vi "WPI_CameraSet White Balance.vi"(8 "error in (no error)":errorcluster, 9 "Color Temp (K)":dbl, 10 "White Balance":T2, 11 "CameraDevRef":T1={"Camera Address"="192.168.0.90", "CameraStatus"={"status"=FALSE, "code"=0, "source"=""}}) -> (0 "error out":errorcluster, 3 "CameraDevRef Out":T1)   [LabVIEW 2017]
doc: "Specifies the white balance setting of the camera you specify.\n\nThis software is licensed. Open the labview\\readme\\WPI Robotics Library Open Source License.txt file for more information."
uses:
  <vilib>/Rock Robotics/WPI/Camera/WPI_CameraWhite Balance Values.ctl
  <vilib>/Rock Robotics/WPI/Camera/WPI_CameraDevRef.ctl
  <vilib>/Rock Robotics/WPI/Camera/WPI_CameraSettings Operations.ctl
  <vilib>/userdefined/High Color/IMAQdx.ctl
  <resource>/objmgr/imaqdx.rc
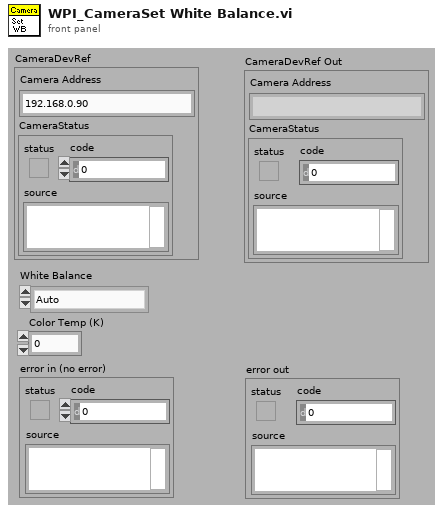
[diagram p1: front panel]
types:
  T1 = typedef "WPI_CameraDevRef.ctl" = cluster{"Camera Address":string, "CameraStatus":errorcluster}
  T2 = typedef "WPI_CameraWhite Balance Values.ctl" = enum16{"Auto", "Fixed indoor", "Fixed outdoor 1", "Fixed outdoor 2", "Fixed fluorescent 1", "Fixed fluorescent 2", "Hold current", "Custom"}
  T3 = typedef "WPI_CameraSettings Operations.ctl" = enum16{"Udate FPS", "Update Compression", "Update Size", "Update White Balance", "Update Brightness", "Update Sharpness", "Update Exposure", "Update Exposure Value", "Update Color Level", "Update Exp Priority", "Update Color Enable", "Update JPG", "Update MJPG", "Read and Clear", "Read", "Init"}
  T4 = typedef "IMAQdx.ctl" = refnum<k21>
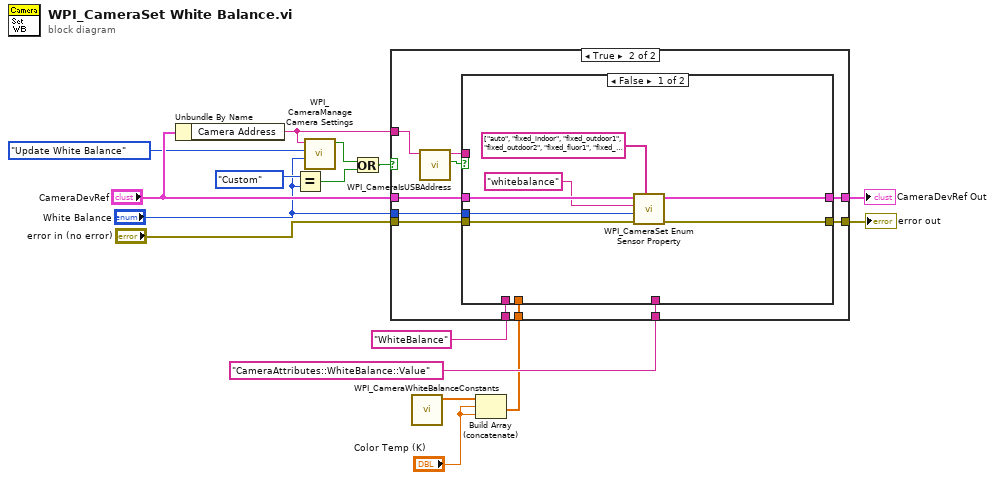
[diagram p0: block diagram]
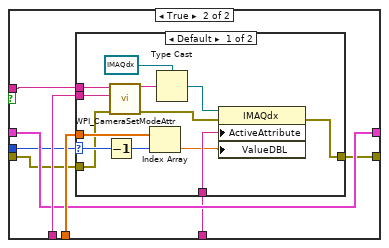
[diagram p3: hidden frame]
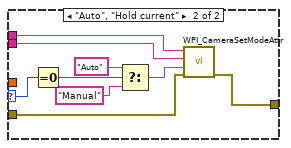
[diagram p4: hidden frame]
diagram:
  n1 = Unbundle By Name("CameraDevRef") -> ("Camera Address"=w11:string)
  n2 = Equal?(x=WPI_CameraWhite_Balance_Values."Custom" ("White Balance"), y="White Balance") -> (x = y?=w3:bool)
  n3 = call <vilib>:"WPI_CameraManage Camera Settings.vi"("Value"="White Balance", "Operation"=WPI_CameraSettings_Operations."Update White Balance", "Camera IP"=w11) -> ("Changed"=w2:bool)  [unwired: 7 in, 1 out]
  n4 = Or(x=w2, y=w3) -> (x .or. y?=w1:bool)
  n5 = call <vilib>:"WPI_CameraWhiteBalanceConstants.vi"() -> ("Color Temps (K)"=w8:dbl[])  [unwired: 11 in]
  n6 = Build Array (concatenate)(w8, "Color Temp (K)", "Color Temp (K)") -> (w7:dbl[])
  n7 = case shown="True" w1 {
    tunnel: [w18 w29] -> w16
    tunnel: [w17 w28] -> w15
    tunnel: "error in (no error)" -> [w17 w27]
    tunnel: "CameraDevRef" -> [w18 w25]
    tunnel: "White Balance" -> [_ w26]
    tunnel: w11 -> [_ w22]
    tunnel: "WhiteBalance" -> [_ w21]
    tunnel: w7 -> [_ w20]
    tunnel: "CameraAttributes::WhiteBalance::Value" -> [_ w19]
    frame False {
    }
    frame True {
      n8 = call <vilib>:"WPI_CameraIsUSBAddress.vi"("Camera Address In"=w22) -> ("USB?"=w24:bool, "Camera Address Out"=w23:string)  [unwired: 8 in, 1 out]
      n9 = case shown="False" w24 {
        tunnel: [w36 w42] -> w29
        tunnel: [w35 w37] -> w28
        tunnel: w27 -> [w34 w38]
        tunnel: w26 -> [w33 w41]
        tunnel: w25 -> [w32 w42]
        tunnel: w23 -> [_ w39]
        tunnel: w21 -> [_ w44]
        tunnel: w20 -> [_ w43]
        tunnel: w19 -> [_ w40]
        frame False {
          n10 = call <vilib>:"WPI_CameraSet Enum Sensor Property.vi"("Strings"=string[] ["auto", "fixed_indoor", "fixed_outdoor1", "fixed_outdoor2", "fixed_fluor1", "fixed_fluor2", "hold", "fixed_fluor", "fixed_outdoor"] ("Array"), "error in (no error)"=w34, "Value"=w33, "Property Name"="whitebalance", "CameraDevRef"=w32) -> ("error out"=w35:errorcluster, "CameraDevRef Out"=w36:T1)  [unwired: 5 out]
        }
        frame True {
          n11 = case shown="Default" w41 {
            selector: w41 -> [w56 w64]
            tunnel: w39 -> [w52 w60]
            tunnel: w44 -> [w51 w61]
            tunnel: w43 -> [w57 _]
            tunnel: w40 -> [w54 _]
            tunnel: w38 -> [w46 w59]
            tunnel: [w47 w58] -> w37
            frame Default {
              n12 = Decrement(x=w56) -> (x-1=w55:T2)
              n13 = call <vilib>:"WPI_CameraSetModeAttr.vi"("error in (no error)"=w46, "Attr String"=w51, "Camera Address In"=w52) -> ("error out"=w45:errorcluster, "Camera Address Out"=w50:string)  [unwired: 7 in]
              n14 = Index Array(array=w57, index=w55) -> (element=w53:dbl)
              n15 = Type Cast(type=T4 refnum ("Session In"), x=w50) -> (*(type *) &x=w49:T4)
              n16 = property class="IMAQdx"(reference=w49, error in=w45, "ActiveAttribute"=w54, "ValueDBL"=w53) -> (error out=w47:errorcluster)  [unwired: 1 out]
            }
            frame "Auto", "Hold current" {
              n17 = Equal To 0?(x=w64) -> (x = 0?=w63:bool)
              n18 = Select(t="Auto", s=w63, f="Manual") -> (s? t:f=w62:string)
              n19 = call <vilib>:"WPI_CameraSetModeAttr.vi"("error in (no error)"=w59, "Value"=w62, "Attr String"=w61, "Camera Address In"=w60) -> ("error out"=w58:errorcluster)  [unwired: 6 in, 1 out]
            }
          }
        }
      }
    }
  }
  "CameraDevRef Out" <- w16
  "error out" <- w15
